vi "RSZVB Select More Wave Quantities With Detector.vi"(0 "VISA session":refnum<visa-resource-name>, 1 "Wave Quantity Port Number (1)":i32=1, 2 "Wave Quantity Type (0: a)":i32(ring) items=["a", "b"], 3 "Detector (0: RMS)":i32(ring) items=["RMS", "Peak", "Average"], 5 "Channel (1)":i32=1, 9 "Trace Name (Trc1)":string="Trc1", 11 "error in (no error)":errorcluster {"code" format="%.0x"}, 12 "Source Port (1: Port 1)":i32=1, 14 "Observation Time (0.01)":dbl=0.01 format="%.2f") -> (4 "dup VISA session":refnum<visa-resource-name>, 15 "error out":errorcluster {"code" format="%.0x"})   [LabVIEW 2011]
doc: "This VI select arbitrary wave quantities with detector, e.g. for different detectors and source ports or more than 2 ports, frequency offsets, or mixed mode measurements.\n\nAssigns a measurement parameter to an existing trace or creates a trace and assigns a channel number, a name and a measurement parameter to it. The trace is not displayed.\n\nThe notation for wave quantities and the VIality of the More Wave Quantities is analogous to the definition of S-parameters.\n\nRemote-control command(s):\nCALCulate<Ch>:PARameter:SDEFine '<string>', 'A1D1SAM' | 'B1D1RMS' | 'B2D1PEAK' | 'A2D2SAM' | 'B1D2RMS' | ...\nCALCulate<Ch>:PARameter:MEASure '<string>', 'A1D1SAM' | 'B1D1RMS' | 'B2D1PEAK' | 'A2D2SAM' | 'B1D2RMS' | ...\n[SENSe<Ch>:]SWEep:DETector:TIME"
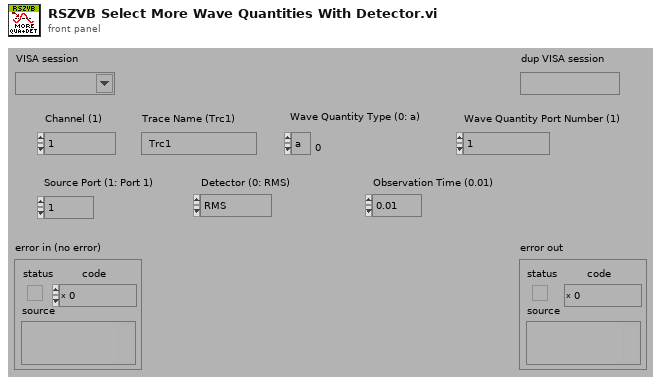
[diagram p1: front panel]
types:
  T1 = cluster{"Error Checking (T: On)":bool, "Installed Options":string[], "Data Valid?":bool, "Ports":i32, "Model":string[], "Option Checking (T: On)":bool}
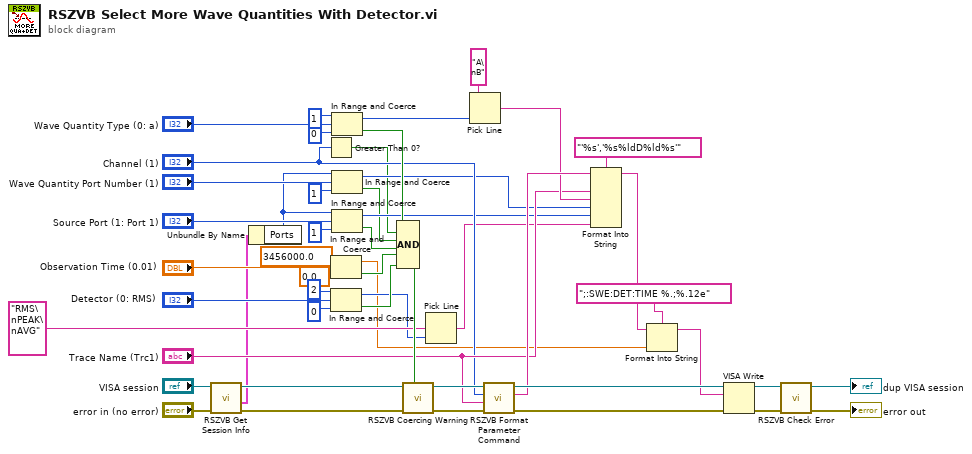
[diagram p0: block diagram]
diagram:
  n1 = call "RSZVB Get Session Info.vi"("error in (no error)"="error in (no error)", "VISA session"="VISA session") -> ("error out"=w4:errorcluster, "Session Info"=w2:T1, "dup VISA session"=w3:refnum<visa-resource-name>)  [unwired: 7 in]
  n2 = Unbundle By Name(w2) -> ("Ports"=w1:i32)
  n3 = Greater Than 0?(x="Channel (1)") -> (x > 0?=w24:bool)
  n4 = In Range and Coerce(upper limit=3456000.0, x="Observation Time (0.01)", lower limit=0.0) -> (coerced(x)=w8:dbl, In Range?=w12:bool)
  n5 = In Range and Coerce(upper limit=2, x="Detector (0: RMS)", lower limit=0) -> (coerced(x)=w9:i32, In Range?=w11:bool)
  n6 = In Range and Coerce(upper limit=1, x="Wave Quantity Type (0: a)", lower limit=0) -> (coerced(x)=w39:i32, In Range?=w37:bool)
  n7 = In Range and Coerce(upper limit=w1, x="Wave Quantity Port Number (1)", lower limit=1) -> (coerced(x)=w26:i32, In Range?=w23:bool)
  n8 = In Range and Coerce(upper limit=w1, x="Source Port (1: Port 1)", lower limit=1) -> (coerced(x)=w25:i32, In Range?=w36:bool)
  n9 = Compound Arithmetic op=AND(w37, w24, w23, w36, w12, w11) -> (w46:bool)
  n10 = call "RSZVB Coercing Warning.vi"("In Range?"=w46, "error in (no error)"=w4, "VISA session"=w3) -> ("error out"=w44:errorcluster, "dup VISA session"=w43:refnum<visa-resource-name>)  [unwired: 7 in]
  n11 = Pick Line(multi-line string="RMS\nPEAK\nAVG", line index=w9) -> (output string=w10:string)  [unwired: 1 in]
  n12 = Pick Line(multi-line string="A\nB", line index=w39) -> (output string=w38:string)  [unwired: 1 in]
  n13 = call "RSZVB Format Parameter Command.vi"("error in (no error)"=w44, "Trace Name (Trc1)"="Trace Name (Trc1)", "Channel (1)"="Channel (1)", "VISA session"=w43) -> ("error out"=w45:errorcluster, "Buffer"=w41:string, "dup VISA session"=w42:refnum<visa-resource-name>)  [unwired: 5 in]
  n14 = Format Into String(format string="'%s','%s%ldD%ld%s'", initial string=w41, "Trace Name (Trc1)", w38, w26, w25, w10) -> (resulting string=w14:string)  [unwired: 1 in, 1 out]
  n15 = Format Into String(format string=";:SWE:DET:TIME %.;%.12e", initial string=w14, w8) -> (resulting string=w13:string)  [unwired: 1 in, 1 out]
  n16 = VISA Write(VISA resource name=w42, write buffer=w13, error in (no error)=w45) -> (VISA resource name out=w47:refnum<visa-resource-name>, error out=w48:errorcluster)  [unwired: 1 out]
  n17 = call "RSZVB Check Error.vi"("error in (no error)"=w48, "VISA session"=w47) -> ("error out"=→"error out":errorcluster, "dup VISA session"=→"dup VISA session":refnum<visa-resource-name>)  [unwired: 8 in]
